vi "Pulse.vi"(0 "Data in":T1, 1 "error in":errorcluster) -> (2 "Data out":T1, 3 "error out":errorcluster, 4 "Ran?":bool)   [LabVIEW 2017, in "Steps.lvlib"]
uses:
  Steps.lvlib
  Type_Defs/Data.ctl
  Type_Defs/Diagnostics.ctl
  Type_Defs/Systems.ctl
panel:
  out "Helical":dbl(graph)
  out "Toroidal":dbl(graph)
  in  "Step Back":bool
  in  "Continue":bool
  # "Verify that the pulse is correct."
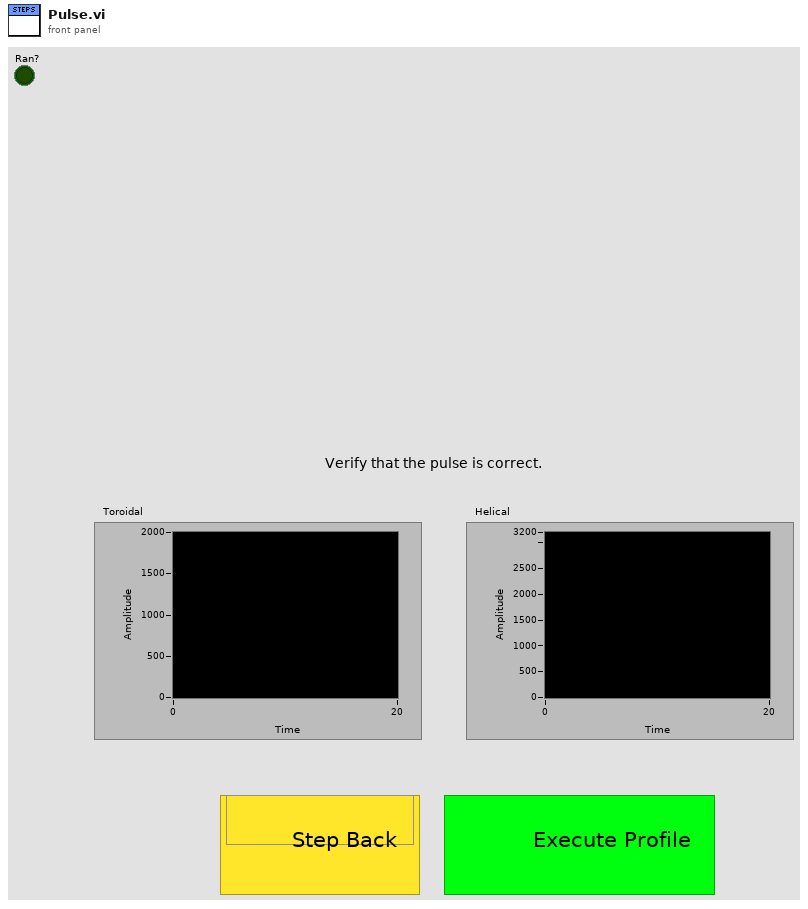
[diagram p1: front panel]
types:
  T1 = typedef "Data.ctl" = cluster{"User Name":string, "Experiment Number":i32, "Start Time":timestamp, "Data":dbl[], "Step Number":i32, "Step Instructions":string, "Diagnostics":T2, "Experiment Purpose":string, "Experiment State":enum16{"Off", "Setting Up", "Ready", "In Progress", "Shutting Down"}, "Systems":T3, "Vacuum Pressure":dbl, "Fieldpoints":cluster{"System Boolean Fieldpoints":cluster{"Compressed Air":refnum<k21>, "T-20kV Power Switch":refnum<k21>, "T-Rectifier":refnum<k21>, "Engage Interlock":refnum<k21>, "Ventilator":refnum<k21>, "Magnetron":refnum<k21>, "H-20kV Power Switch":refnum<k21>, "H-Rectifier":refnum<k21>, "Main Water Pump":refnum<k21>, "WEGA Water Pump":refnum<k21>, "Gas Inlet Valves":refnum<k21>}, "Step Fieldpoints":cluster{"Exhaust Ventillator":refnum<k21>, "Compressed Air":refnum<k21>, "Water Pressure":refnum<k21>, "Interlock":refnum<k21>, "Toroidal Power Supply 1":refnum<k21>, "Toroidal Power Supply 2":refnum<k21>, "Toroidal Rectifier":refnum<k21>, "Helical Power Supply":refnum<k21>, "Helical Rectifier":refnum<k21>, "6kW Magnetron Standby":refnum<k21>, "20kW Magnetron Standby":refnum<k21>}}, "Pressure History":cluster{"Seconds into Experiment":i32[], "Pressure Data":dbl[]}, "Time Computer Control":dbl[], "Toroidal Voltage Computer Control":dbl[], "Helical Voltage Computer Control":dbl[], "Toroidal Current":dbl[], "Toroidal Voltage":dbl[], "Toroidal Current Set Point":dbl[], "Helical Current Set Point":dbl[], "Helical Voltage":dbl[], "Helical Current":dbl[], "Experiment Folder":path, "Run Another Shot?":bool}
  T2 = typedef "Diagnostics.ctl" = cluster{"Langmuir Probe":bool, "Rogowski 1":bool, "Rogowski 2":bool, "Rogowski 3":bool, "B-dot 1":bool, "B-dot 2":bool}
  T3 = typedef "Systems.ctl" = cluster{"Compressed Air":bool, "T-20kV Power Switch":bool, "T-Rectifier":bool, "Engage Interlock":bool, "Ventilator":bool, "Magnetron":bool, "H-20kV Power Switch":bool, "H-Rectifier":bool, "Main Water Pump":bool, "WEGA Water Pump":bool, "Gas Inlet Valves":bool}
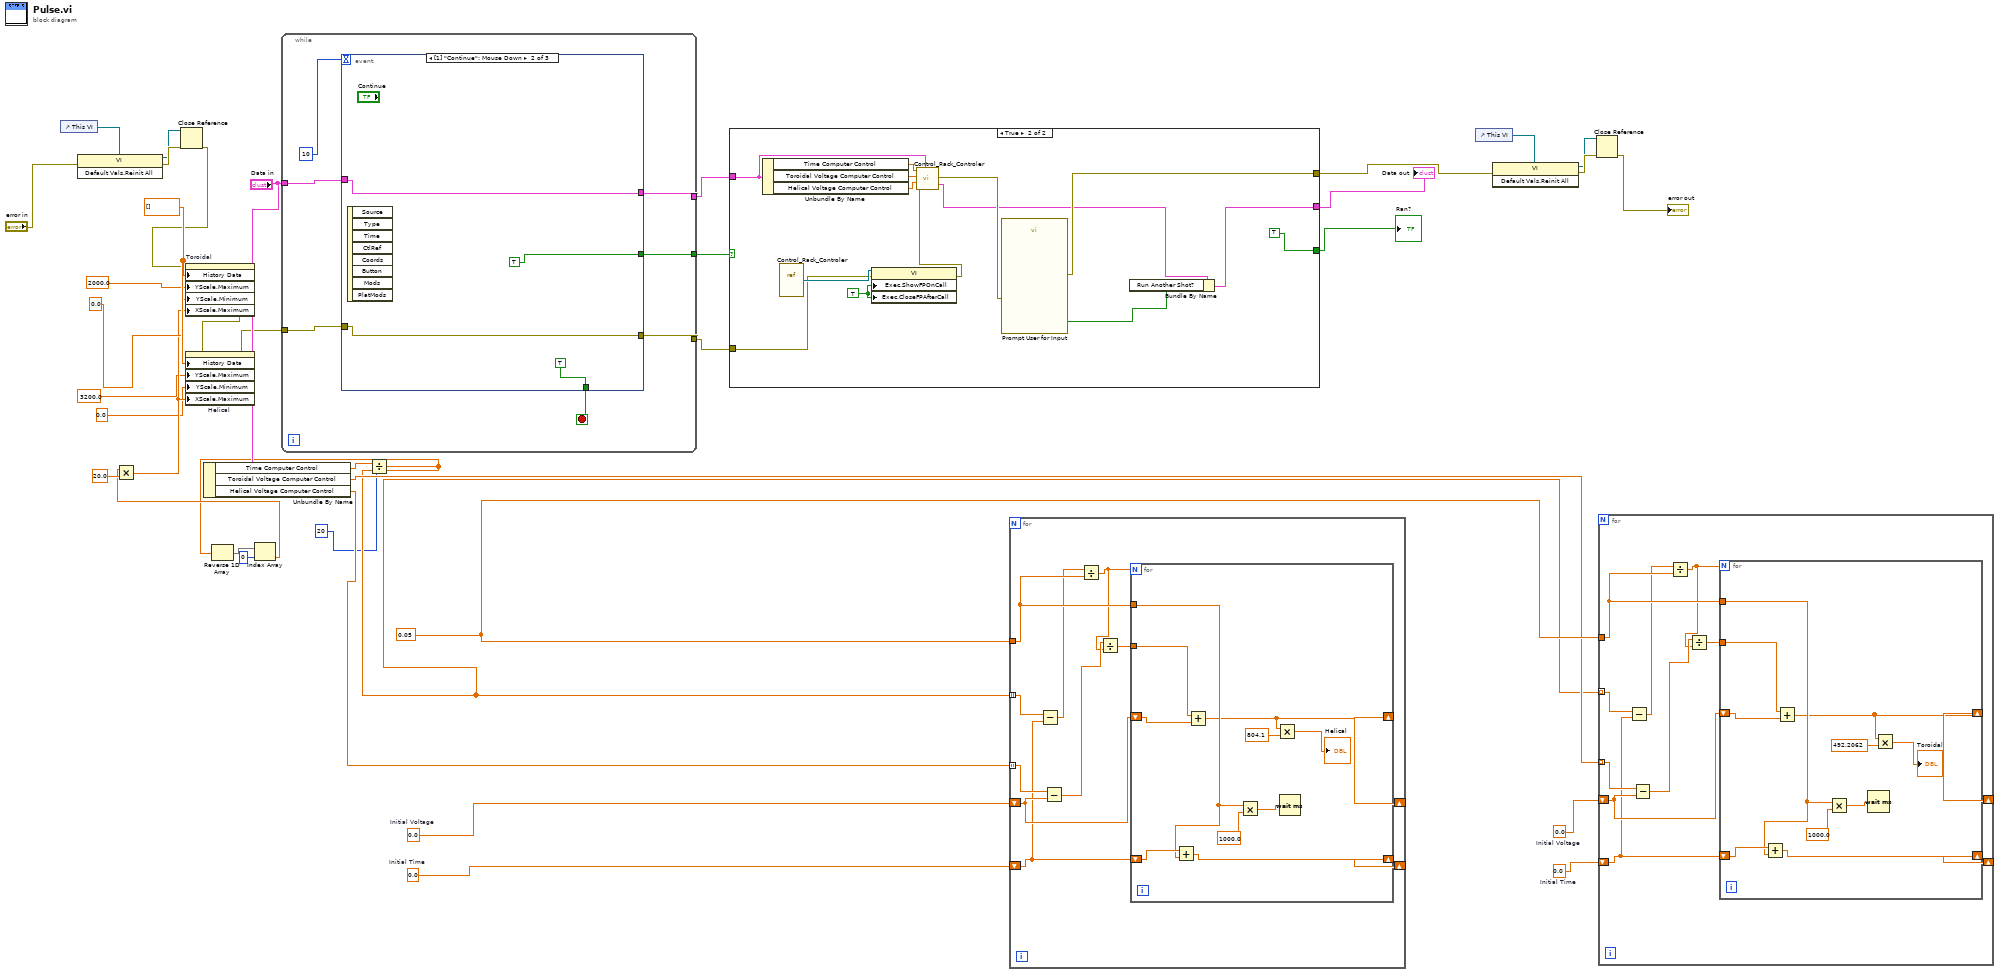
[diagram p0: block diagram]
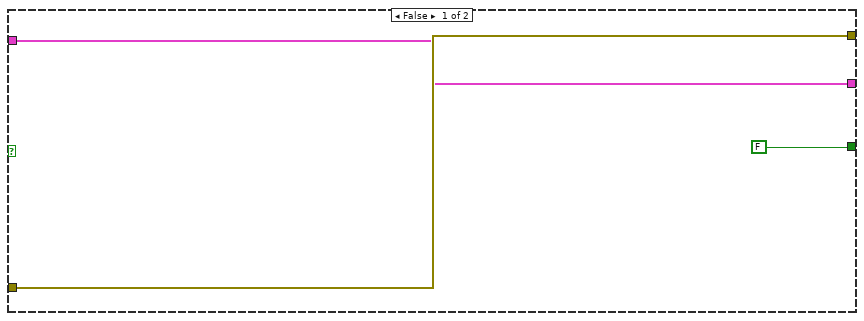
[diagram p2: hidden frame]
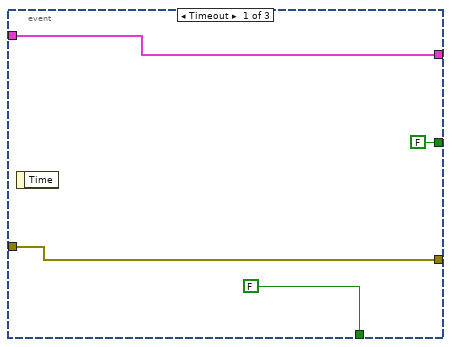
[diagram p3: hidden frame]
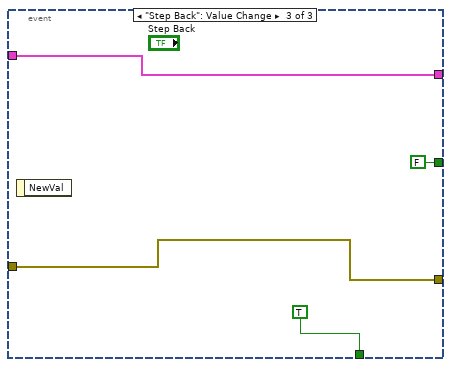
[diagram p4: hidden frame]
diagram:
  w28 = dbl[] [] ("History Data")
  w33 = 0.05 ("Timestep (in seconds, keep above 1/20s)")
  w35 = 0.0  # Initial Time
  w34 = 0.0  # Initial Voltage
  w36 = 0.0  # Initial Time
  w37 = 0.0  # Initial Voltage
  n1 = control-ref of="This VI"() -> (w15:refnum<vi>)
  n2 = invoke class="VI" method="Default Vals.Reinit All"(reference=w15, error in="error in") -> (reference out=w11:refnum<vi>, error out=w12:errorcluster)  [unwired: 1 in, 1 out]
  n3 = Close Reference(reference=w11, error in (no error)=w12) -> (error out=w14:errorcluster)
  n4 = Unbundle By Name("Data in") -> ("Time Computer Control"=w19:dbl[], "Toroidal Voltage Computer Control"=w31:dbl[], "Helical Voltage Computer Control"=w32:dbl[])
  n5 = Divide(x=w19, y=20 ("Time Computer Control")) -> (x/y=w20:dbl[])
  n6 = Reverse 1D Array(array=w20) -> (reversed array=w27:dbl[])
  n7 = Index Array(array=w27, index=0) -> (element=w22:dbl)
  n8 = Multiply(x=w22, y=20.0) -> (x*y=w21:dbl)
  n9 = property on="Toroidal" class="WFChart (strict)"(error in=w14, "History Data"=w28, "YScale.Maximum"=2000.0 ("Y Scale.Range:Maximum"), "YScale.Minimum"=0.0 ("Y Scale.Range:Maximum"), "XScale.Maximum"=w21) -> (error out=w30:errorcluster)  [unwired: 1 in, 1 out]
  n10 = property on="Helical" class="WFChart (strict)"(error in=w30, "History Data"=w28, "YScale.Maximum"=3200.0 ("Y Scale.Range:Maximum"), "YScale.Minimum"=0.0 ("Y Scale.Range:Maximum"), "XScale.Maximum"=w21) -> (error out=w29:errorcluster)  [unwired: 1 in, 1 out]
  n11 = while {
    tunnel: w29 -> [w45]
    tunnel: [w44] -> w5
    tunnel: [w42] -> w4
    tunnel: "Data in" -> [w41]
    tunnel: [w39] -> w6
    stop <- w43 stop-if-true
    n12 = event shown="[1] \"Continue\": Mouse Down" {
      selector: _ -> [_ _ _]
      dyn-events: _ -> [_ _ _]
      timeout: 10 -> [_ _ _]
      tunnel: w45 -> [w48 w50 w55]
      tunnel: [w48 w50 w55] -> w44
      tunnel: [FALSE TRUE TRUE] -> w43
      tunnel: [w47 w51 w56] -> w42
      tunnel: w41 -> [w47 w51 w56]
      tunnel: [FALSE TRUE FALSE] -> w39
      event Timeout {
        n13 = event-data() -> ()  [unwired: 1 in, 1 out]
      }
      event "Continue": Mouse Down {
        n14 = event-data() -> ()  [unwired: 1 in, 8 out]
      }
      event "Step Back": Value Change {
        n15 = event-data() -> ()  [unwired: 1 in, 1 out]
      }
    }
  }
  n16 = case shown="True" w6 {
    tunnel: [w59 w69] -> w2
    tunnel: [w58 w67] -> w3
    tunnel: [FALSE TRUE] -> w1
    tunnel: w4 -> [w58 w61]
    tunnel: w5 -> [w59 w65]
    frame False {
    }
    frame True {
      w74 = TRUE ("Execution:Show Front Panel On Call")
      n17 = Unbundle By Name(w61) -> ("Time Computer Control"=w64:dbl[], "Toroidal Voltage Computer Control"=w62:dbl[], "Helical Voltage Computer Control"=w63:dbl[])
      n18 = vi-ref "Control_Rack_Controler.vi"() -> (w72:refnum<vi>)
      n19 = property class="VI"(reference=w72, error in=w65, "Exec.ShowFPOnCall"=w74, "Exec.CloseFPAfterCall"=w74) -> (error out=w73:errorcluster)  [unwired: 1 out]
      n20 = call "Control_Rack_Controler.vi"("Times"=w64, "Voltages Toroidal (Keep below |10|)"=w62, "Voltages Helical (Keep below |10|)"=w63, "error out"=w73, "Data in"=w61) -> ("error out 2"=w70:errorcluster, "Data out"=w68:T1)
      n21 = call "Prompt User for Input"("error in (no error)"=w70) -> ("Run New Shot"=w71:bool, "error out"=w69:errorcluster)  [unwired: 16 in, 1 out]
      n22 = Bundle By Name(cluster=w68, "Run Another Shot?"=w71) -> (w67:T1)
    }
  }
  "Data out" <- w3
  "Ran?" <- w1
  n23 = for {
    tunnel: w32 -> [w85] mode=indexing
    tunnel: w20 -> [w78] mode=indexing
    tunnel: w33 -> [w80]
    shift-right: [w81] -> _
    shift-left: w37 -> [w84]
    shift-right: [w79] -> _
    shift-left: w36 -> [w77]
    n24 = Subtract(x=w78, y=w77) -> (x-y=w76:dbl)
    n25 = Subtract(x=w85, y=w84) -> (x-y=w83:dbl)
    n26 = Divide(x=w76, y=w80) -> (x/y=w75:dbl)
    n27 = Divide(x=w83, y=w75) -> (x/y=w82:dbl)
    n28 = for {
      N: w75 -> [_]
      shift-right: [w87] -> w81
      shift-left: w84 -> [w95]
      tunnel: w82 -> [w94]
      tunnel: w80 -> [w91]
      shift-right: [w89] -> w79
      shift-left: w77 -> [w93]
      n29 = Add(x=w93, y=w91) -> (x+y=w89:dbl)
      n30 = Add(x=w94, y=w95) -> (x+y=w87:dbl)
      n31 = Multiply(x=w91, y=1000.0) -> (x*y=w92:dbl)
      n32 = Multiply(x=w87, y=804.1) -> (x*y=→"Helical":dbl)
      n33 = Wait (ms)(milliseconds to wait=w92) -> ()  [unwired: 1 out]
    }
  }
  n34 = control-ref of="This VI"() -> (w10:refnum<vi>)
  n35 = invoke class="VI" method="Default Vals.Reinit All"(reference=w10, error in=w2) -> (reference out=w8:refnum<vi>, error out=w9:errorcluster)  [unwired: 1 in, 1 out]
  n36 = Close Reference(reference=w8, error in (no error)=w9) -> (error out=→"error out":errorcluster)
  n37 = for {
    tunnel: w31 -> [w106] mode=indexing
    tunnel: w20 -> [w99] mode=indexing
    tunnel: w33 -> [w101]
    shift-right: [w102] -> _
    shift-left: w34 -> [w105]
    shift-right: [w100] -> _
    shift-left: w35 -> [w98]
    n38 = Subtract(x=w99, y=w98) -> (x-y=w97:dbl)
    n39 = Subtract(x=w106, y=w105) -> (x-y=w104:dbl)
    n40 = Divide(x=w97, y=w101) -> (x/y=w96:dbl)
    n41 = Divide(x=w104, y=w96) -> (x/y=w103:dbl)
    n42 = for {
      N: w96 -> [_]
      shift-right: [w107] -> w102
      shift-left: w105 -> [w116]
      tunnel: w103 -> [w115]
      tunnel: w101 -> [w112]
      shift-right: [w110] -> w100
      shift-left: w98 -> [w114]
      n43 = Add(x=w114, y=w112) -> (x+y=w110:dbl)
      n44 = Add(x=w115, y=w116) -> (x+y=w107:dbl)
      n45 = Multiply(x=w112, y=1000.0) -> (x*y=w113:dbl)
      n46 = Wait (ms)(milliseconds to wait=w113) -> ()  [unwired: 1 out]
      n47 = Multiply(x=w107, y=492.2062) -> (x*y=→"Toroidal":dbl)
    }
  }
